vi "Test Data Graph02.vi"() -> ()   [LabVIEW 2020]
uses:
  <vilib>/measure/NI_MABase.lvlib
panel:
  in  "Load":bool
  out "XY":cluster{timestamp[], dbl[]}[](graph)
  in  "P1":dbl(slide) scale=3772664021.7079873..3772664023.307987 scale format="%<%m/%d %H:%M:%S>T"
  in  "P2":dbl(slide) scale=3772664021.7079873..3772664023.307987 scale format="%<%m/%d %H:%M:%S>T"
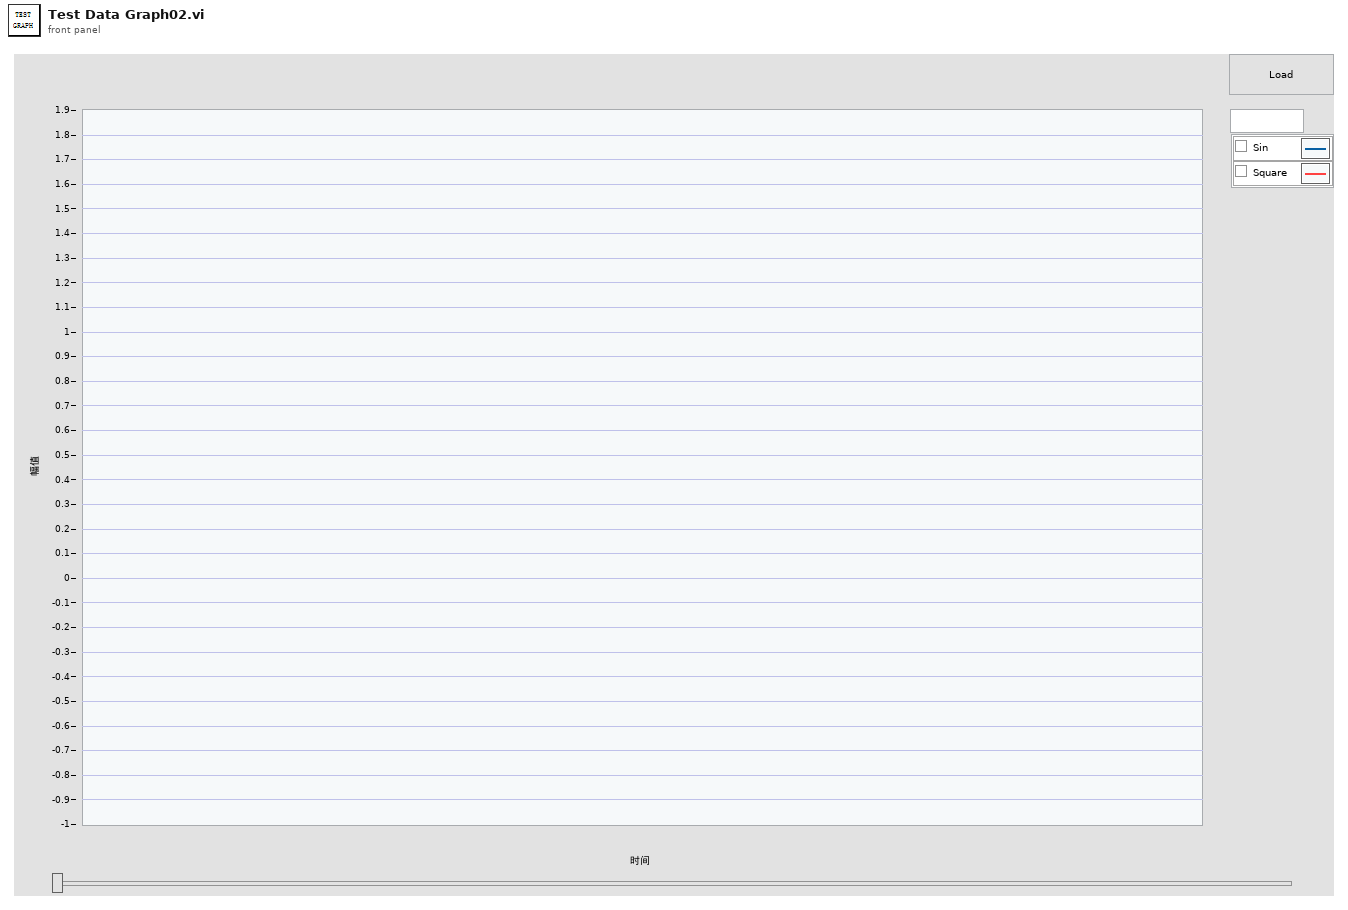
[diagram p1: front panel]
types:
  T1 = cluster{"XY":refnum<vi>, "Maxpoint":i32, "P1":refnum<vi>, "P2":refnum<vi>, "Range":cluster{"IStart":dbl, "CRange":dbl, "IRange":dbl, "CStart":dbl, "Stop":dbl}, "Data":map{string, cluster{"Init":waveform(dbl), "Current":waveform(dbl)}}, "ID":string[]}
  T2 = map{string, cluster{"Init":waveform(dbl), "Current":waveform(dbl)}}
  T3 = cluster{"signal out":waveform(dbl), "signal out":waveform(dbl)}
  T4 = typedef "LVRangeTypeDef.ctl" = cluster{"Minimum":dbl, "Maximum":dbl, "Increment":dbl, "Minor Increment":dbl, "Start":dbl}
  T5 = cluster{"Init":waveform(dbl), "Current":waveform(dbl)}
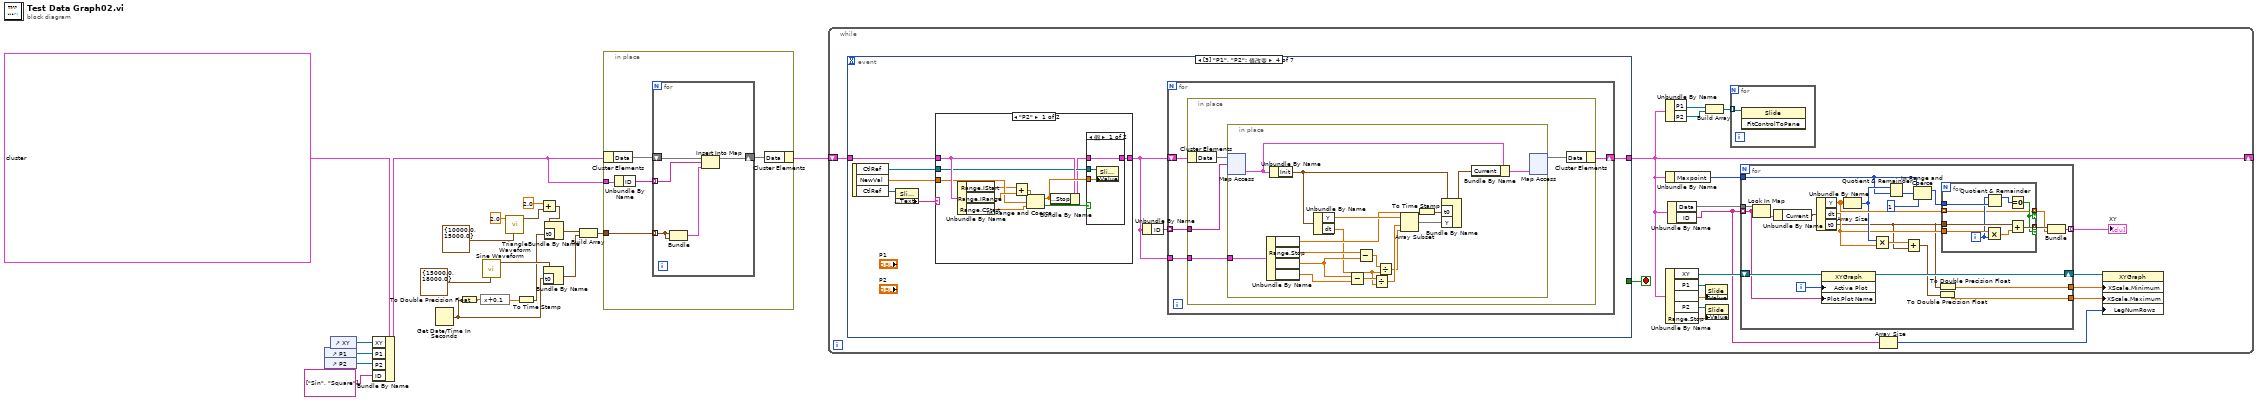
[diagram p0: block diagram]
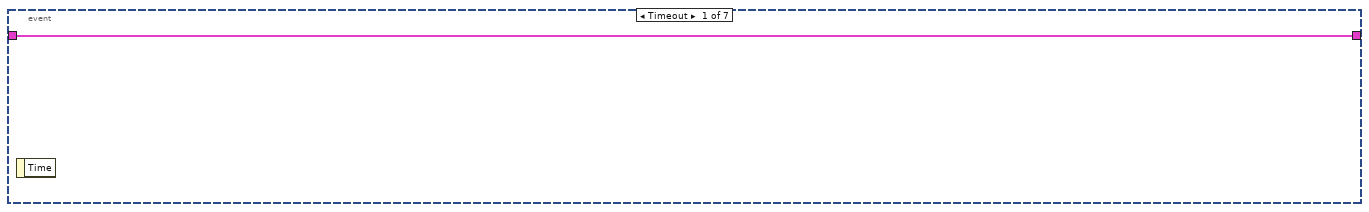
[diagram p2: hidden frame]
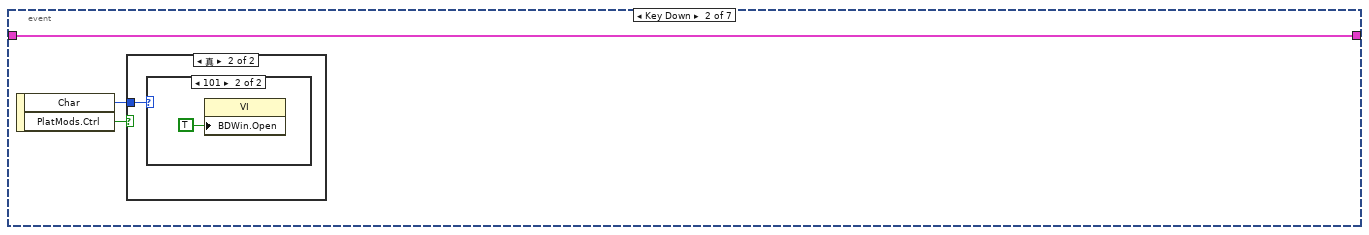
[diagram p3: hidden frame]
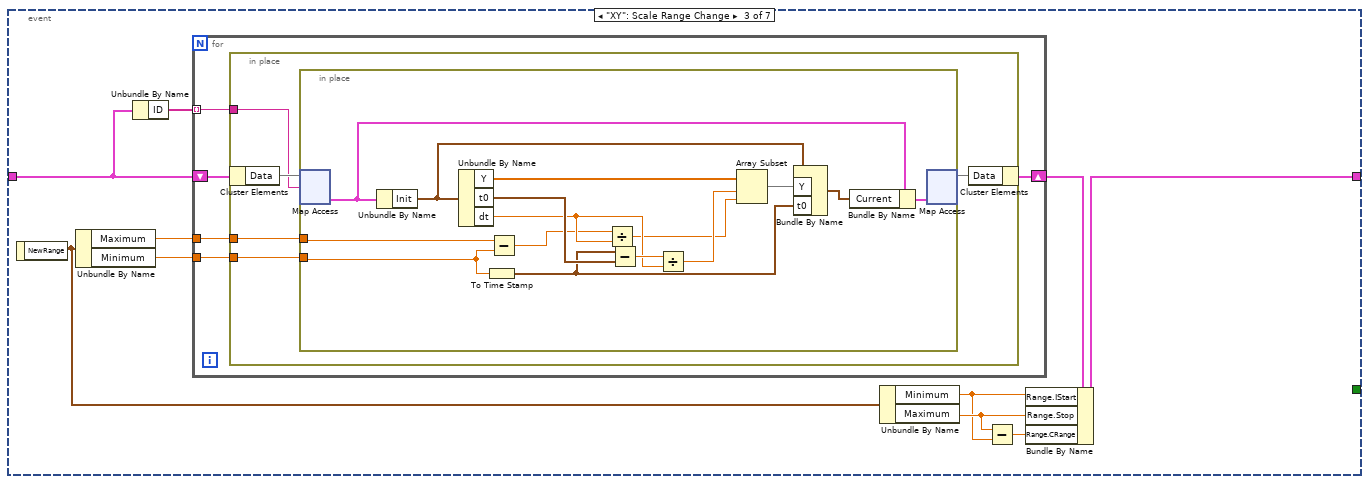
[diagram p6: hidden frame]
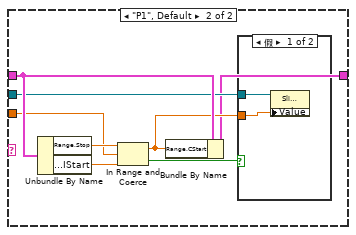
[diagram p8: hidden frame]
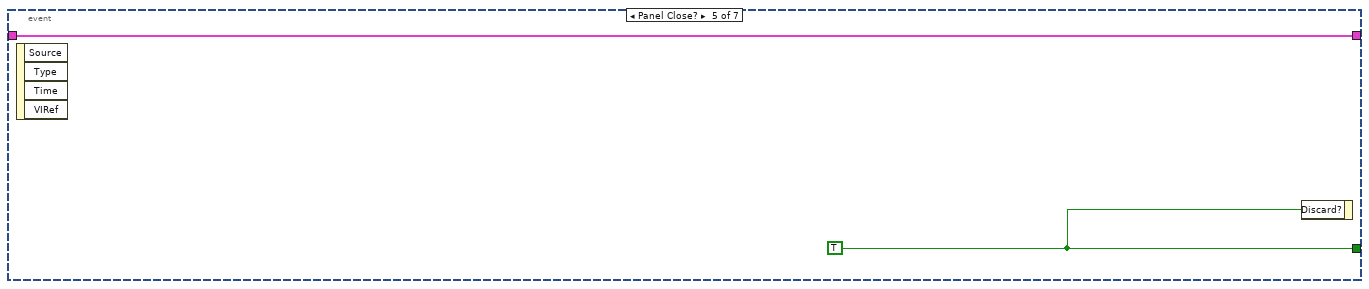
[diagram p10: hidden frame]
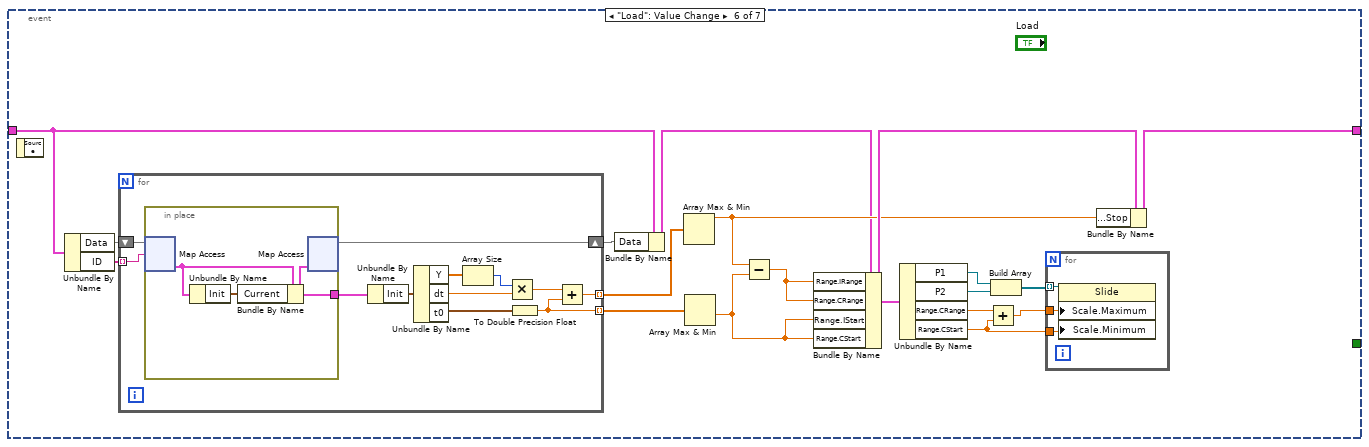
[diagram p11: hidden frame]
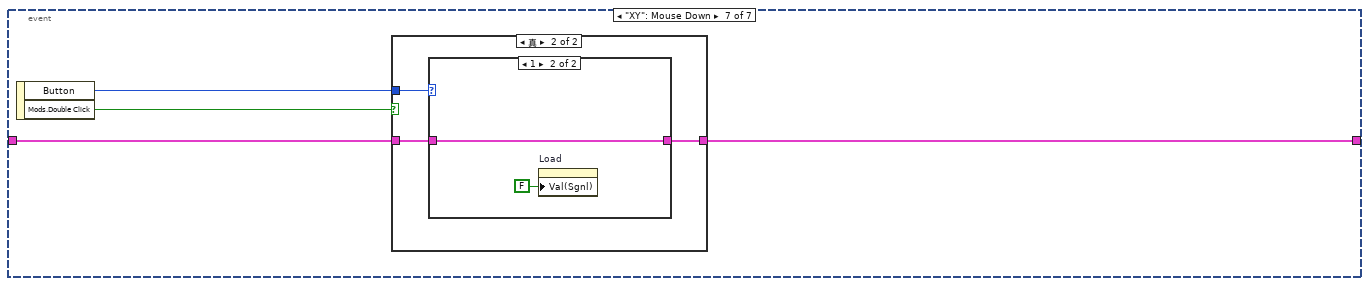
[diagram p12: hidden frame]
diagram:
  n1 = control-ref of="P1"() -> (w19:refnum<vi>)
  n2 = control-ref of="P2"() -> (w18:refnum<vi>)
  n3 = control-ref of="XY"() -> (w20:refnum<vi>)
  n4 = Bundle By Name(cluster=T1 {"XY"=refnum, "Maxpoint"=5000, "P1"=refnum, "P2"=refnum, "Range"={"IStart"=0.0, "CRange"=0.0, "IRange"=0.0, "CStart"=0.0, "Stop"=0.0}, "Data"={}, "ID"=[]}, "XY"=w20, "P1"=w19, "P2"=w18, "ID"=string[] ["Sin", "Square"]) -> (w10:T1)
  n5 = Get Date/Time In Seconds() -> (seconds since 1Jan1904=w3:timestamp)
  n6 = To Double Precision Float(number=w3) -> (double precision float=w16:dbl)
  n7 = expression code="x+0.1"(w16) -> (w17:dbl)
  n8 = call <vilib>:"Sine Waveform.vi"("sampling info"=cluster{"Fs":dbl, "#s":dbl} {"Fs"=15000.0, "#s"=18000.0}) -> ("signal out"=w15:waveform(dbl))  [unwired: 9 in, 1 out]
  n9 = call <vilib>:"Triangle Waveform.vi"("sampling info"=cluster{"Fs":dbl, "#s":dbl} {"Fs"=10000.0, "#s"=15000.0}, "frequency"=2.0) -> ("signal out"=w6:waveform(dbl))  [unwired: 8 in, 1 out]
  n10 = To Time Stamp(1:w17) -> (0:w2:timestamp)
  n11 = Add(x=2.0, y=w6) -> (x+y=w4:waveform(dbl))
  n12 = Bundle By Name(cluster=w15, "t0"=w3) -> (w8:waveform(dbl))
  n13 = Bundle By Name(cluster=w4, "t0"=w2) -> (w9:waveform(dbl))
  n14 = Build Array(w9, w8) -> (w7:waveform(dbl)[])
  n15 = in-place {
    in-place-border: w10 -> [w25]
    in-place-border: w7 -> [w23]
    n16 = in-place-cluster #1(w10) -> ("Data"=w26:T2)
    n17 = Unbundle By Name(w25) -> ("ID"=w24:string[])
    n18 = for {
      shift-right: [w27] -> w22
      shift-left: w26 -> [w31]
      tunnel: w24 -> [w30] mode=indexing
      tunnel: w23 -> [w29] mode=indexing
      n19 = Bundle("signal out"=w29, "signal out"=w29) -> (w28:T3)  [unwired: 1 in]
      n20 = Insert Into Map(map in=w31, key=w30, value=w28) -> (map out=w27:T2)  [unwired: 2 out]
    }
    n21 = in-place-cluster #1("Data"=w22) -> (w12:T1)
  }
  n22 = while {
    shift-right: [w38] -> _
    shift-left: w12 -> [w48]
    stop <- w49 stop-if-true
    n23 = event shown="[3] \"P1\", \"P2\": 值改变" {
      selector: _ -> [_ _ _ _ _ _ _]
      dyn-events: _ -> [_ _ _ _ _ _ _]
      timeout: _ -> [_ _ _ _ _ _ _]
      tunnel: [_ _ _ _ w182 _ _] -> w49
      tunnel: [w82 w83 w96 w128 w181 w194 w219] -> w38
      tunnel: w48 -> [w82 w83 w94 w130 w181 w192 w220]
      event Timeout {
        n24 = event-data() -> ()  [unwired: 1 in, 1 out]
      }
      event Key Down {
        n25 = event-data() -> ("Char"=w85:i16, "PlatMods.Ctrl"=w84:bool)  [unwired: 1 in]
        n26 = case shown="真" w84 {
          tunnel: w85 -> [_ w86]
          frame False {
          }
          frame True {
            n27 = case shown="101" w86 {
              frame 0, Default {
              }
              frame 101 {
                n28 = property class="VI"("BDWin.Open"=TRUE ("程序框图窗口:打开")) -> ()  [unwired: 2 in, 2 out]
              }
            }
          }
        }
      }
      event "XY": Scale Range Change {
        n29 = event-data() -> ("NewRange"=w91:T4)  [unwired: 1 in]
        n30 = Unbundle By Name(w91) -> ("Maximum"=w95:dbl, "Minimum"=w92:dbl)
        n31 = Unbundle By Name(w94) -> ("ID"=w93:string[])
        n32 = for {
          tunnel: w92 -> [w102]
          tunnel: w95 -> [w101]
          shift-right: [w99] -> w97
          shift-left: w94 -> [w100]
          tunnel: w93 -> [w98] mode=indexing
          n33 = in-place {
            in-place-border: w102 -> [w107]
            in-place-border: w101 -> [w106]
            in-place-border: w98 -> [w103]
            n34 = in-place-cluster #2(w100) -> ("Data"=w105:T2)
            n35 = in-place {
              in-place-border: w107 -> [w121]
              in-place-border: w106 -> [w110]
              n36 = in-place-map #3(w105, w103) -> (w109:T5)  [unwired: 1 in, 1 out]
              n37 = Unbundle By Name(w109) -> ("Init"=w114:waveform(dbl))
              n38 = Unbundle By Name(w114) -> ("Y"=w120:dbl[], "t0"=w122:timestamp, "dt"=w117:dbl)
              n39 = To Time Stamp(1:w121) -> (0:w112:timestamp)
              n40 = Subtract(x=w110, y=w121) -> (x-y=w111:dbl)
              n41 = Divide(x=w111, y=w117) -> (x/y=w115:dbl)
              n42 = Subtract(x=w112, y=w122) -> (x-y=w118:dbl)
              n43 = Divide(x=w118, y=w117) -> (x/y=w116:dbl)
              n44 = Array Subset(array=w120, index=w116, length=w115) -> (w119:dbl[])
              n45 = Bundle By Name(cluster=w114, "Y"=w119, "t0"=w112) -> (w113:waveform(dbl))
              n46 = Bundle By Name(cluster=w109, "Current"=w113) -> (w108:T5)
              n47 = in-place-map #3(w108) -> (w104:T2)  [unwired: 1 in, 2 out]
            }
            n48 = in-place-cluster #2("Data"=w104) -> (w99:T1)
          }
        }
        n49 = Unbundle By Name(w91) -> ("Minimum"=w89:dbl, "Maximum"=w90:dbl)
        n50 = Subtract(x=w90, y=w89) -> (x-y=w88:dbl)
        n51 = Bundle By Name(cluster=w97, "Range.IStart"=w89, "Range.Stop"=w90, "Range.CRange"=w88) -> (w96:T1)
      }
      event "P1", "P2": Value Change {
        n52 = event-data() -> ("CtlRef"=w125:refnum<vi>, "NewVal"=w129:dbl, "CtlRef"=w127:refnum<vi>)  [unwired: 1 in]
        n53 = property class="Slide (严格)"(reference=w127) -> ("Label.Text"=w126:string)  [unwired: 1 in, 2 out]
        n54 = case shown="\"P2\"" w126 {
          tunnel: w130 -> [w161 w178]
          tunnel: w129 -> [w159 w176]
          tunnel: w125 -> [w160 w174]
          tunnel: [w162 w171] -> w123
          frame "P2" {
            n55 = Unbundle By Name(w161) -> ("Range.IStart"=w157:dbl, "Range.IRange"=w164:dbl, "Range.CStart"=w156:dbl)
            n56 = Add(x=w157, y=w164) -> (x+y=w163:dbl)
            n57 = In Range and Coerce(upper limit=w163, x=w159, lower limit=w156) -> (coerced(x)=w166:dbl, In Range?=w165:bool)
            n58 = Bundle By Name(cluster=w161, "Range.Stop"=w166) -> (w158:T1)
            n59 = case shown="假" w165 {
              tunnel: w158 -> [w168 w170]
              tunnel: w166 -> [w169 _]
              tunnel: [w168 w170] -> w162
              tunnel: w160 -> [w167 _]
              frame False {
                n60 = property class="Slide (严格)"(reference=w167, "Value"=w169) -> ()  [unwired: 1 in, 2 out]
              }
              frame True {
              }
            }
          }
          frame "P1", Default {
            n61 = Unbundle By Name(w178) -> ("Range.Stop"=w177:dbl, "Range.IStart"=w175:dbl)
            n62 = In Range and Coerce(upper limit=w177, x=w176, lower limit=w175) -> (coerced(x)=w173:dbl, In Range?=w172:bool)
            n63 = Bundle By Name(cluster=w178, "Range.CStart"=w173) -> (w171:T1)
            n64 = case shown="假" w172 {
              tunnel: w174 -> [w180 _]
              tunnel: w173 -> [w179 _]
              frame False {
                n65 = property class="Slide (严格)"(reference=w180, "Value"=w179) -> ()  [unwired: 1 in, 2 out]
              }
              frame True {
              }
            }
          }
        }
        n66 = Unbundle By Name(w123) -> ("ID"=w124:string[])
        n67 = for {
          shift-right: [w132] -> w128
          shift-left: w123 -> [w134]
          tunnel: w124 -> [w133] mode=indexing
          tunnel: w123 -> [w131]
          n68 = in-place {
            in-place-border: w133 -> [w136]
            in-place-border: w131 -> [w135]
            n69 = in-place-cluster #4(w134) -> ("Data"=w138:T2)
            n70 = in-place {
              in-place-border: w135 -> [w139]
              n71 = in-place-map #5(w138, w136) -> (w141:T5)  [unwired: 1 in, 1 out]
              n72 = Unbundle By Name(w139) -> ("Range.CStart"=w144:dbl, "Range.Stop"=w153:dbl, "Range.CStart"=w143:dbl, "Range.IStart"=w149:dbl)
              n73 = Unbundle By Name(w141) -> ("Init"=w152:waveform(dbl))
              n74 = Unbundle By Name(w152) -> ("Y"=w150:dbl[], "dt"=w142:dbl)
              n75 = Subtract(x=w143, y=w149) -> (x-y=w148:dbl)
              n76 = Subtract(x=w153, y=w143) -> (x-y=w151:dbl)
              n77 = Divide(x=w148, y=w142) -> (x/y=w146:dbl)
              n78 = Divide(x=w151, y=w142) -> (x/y=w145:dbl)
              n79 = Array Subset(array=w150, index=w146, length=w145) -> (w147:dbl[])
              n80 = To Time Stamp(1:w144) -> (0:w155:timestamp)
              n81 = Bundle By Name(cluster=w152, "t0"=w155, "Y"=w147) -> (w154:waveform(dbl))
              n82 = Bundle By Name(cluster=w141, "Current"=w154) -> (w140:T5)
              n83 = in-place-map #5(w140) -> (w137:T2)  [unwired: 1 in, 2 out]
            }
            n84 = in-place-cluster #4("Data"=w137) -> (w132:T1)
          }
        }
      }
      event Panel Close? {
        w182 = TRUE ("放弃？")
        n85 = event-data() -> ()  [unwired: 1 in, 4 out]
        n86 = event-data("Discard?"=w182) -> ()  [unwired: 1 in, 1 out]
      }
      event "Load": Value Change {
        n87 = event-data() -> ()  [unwired: 1 in, 1 out]
        n88 = Unbundle By Name(w192) -> ("Data"=w185:T2, "ID"=w191:string[])
        n89 = for {
          tunnel: w191 -> [w204] mode=indexing
          tunnel: [w206] -> w189 mode=indexing
          tunnel: [w205] -> w190 mode=indexing
          shift-right: [w202] -> w183
          shift-left: w185 -> [w203]
          n90 = in-place {
            in-place-border: [w213] -> w201
            n91 = in-place-map #6(w203, w204) -> (w215:T5)  [unwired: 1 in, 1 out]
            n92 = Unbundle By Name(w215) -> ("Init"=w214:waveform(dbl))
            n93 = Bundle By Name(cluster=w215, "Current"=w214) -> (w213:T5)
            n94 = in-place-map #6(w213) -> (w202:T2)  [unwired: 1 in, 2 out]
          }
          n95 = Unbundle By Name(w201) -> ("Init"=w208:waveform(dbl))
          n96 = Unbundle By Name(w208) -> ("Y"=w211:dbl[], "dt"=w210:dbl, "t0"=w209:timestamp)
          n97 = Array Size(array=w211) -> (size(s)=w212:i32)
          n98 = Multiply(x=w212, y=w210) -> (x*y=w207:dbl)
          n99 = To Double Precision Float(number=w209) -> (double precision float=w206:dbl)
          n100 = Add(x=w207, y=w206) -> (x+y=w205:dbl)
        }
        n101 = Bundle By Name(cluster=w192, "Data"=w183) -> (w184:T1)
        n102 = Array Max & Min(array=w190) -> (max value=w187:dbl)  [unwired: 3 out]
        n103 = Array Max & Min(array=w189) -> (min value=w188:dbl)  [unwired: 3 out]
        n104 = Subtract(x=w187, y=w188) -> (x-y=w186:dbl)
        n105 = Bundle By Name(cluster=w184, "Range.IRange"=w186, "Range.CRange"=w186, "Range.IStart"=w188, "Range.CStart"=w188) -> (w196:T1)
        n106 = Unbundle By Name(w196) -> ("P1"=w199:refnum<vi>, "P2"=w198:refnum<vi>, "Range.CRange"=w197:dbl, "Range.CStart"=w195:dbl)
        n107 = Add(x=w197, y=w195) -> (x+y=w193:dbl)
        n108 = Build Array(w199, w198) -> (w200:refnum<vi>[])
        n109 = for {
          tunnel: w200 -> [w218] mode=indexing
          tunnel: w193 -> [w217]
          tunnel: w195 -> [w216]
          n110 = property class="Slide"(reference=w218, "Scale.Maximum"=w217, "Scale.Minimum"=w216) -> ()  [unwired: 1 in, 2 out]
        }
        n111 = Bundle By Name(cluster=w196, "Range.Stop"=w187) -> (w194:T1)
      }
      event "XY": Mouse Down {
        n112 = event-data() -> ("Button"=w221:u16, "Mods.Double Click"=w222:bool)  [unwired: 1 in]
        n113 = case shown="真" w222 {
          tunnel: w221 -> [_ w226]
          tunnel: [w223 w225] -> w219
          tunnel: w220 -> [w223 w224]
          frame False {
          }
          frame True {
            n114 = case shown="1" w226 {
              tunnel: [w227 w229] -> w225
              tunnel: w224 -> [w227 w229]
              frame 0, Default {
              }
              frame 1 {
                n115 = property on="Load" class="Bool (严格)"("Val(Sgnl)"=FALSE ("值(信号)")) -> ()  [unwired: 2 in, 2 out]
              }
            }
          }
        }
      }
    }
    n116 = Unbundle By Name(w38) -> ("P1"=w39:refnum<vi>, "P2"=w40:refnum<vi>)
    n117 = Unbundle By Name(w38) -> ("Maxpoint"=w45:i32)
    n118 = Unbundle By Name(w38) -> ("XY"=w34:refnum<vi>, "P1"=w44:refnum<vi>, "Range.CStart"=w42:dbl, "P2"=w43:refnum<vi>, "Range.Stop"=w37:dbl)
    n119 = Unbundle By Name(w38) -> ("Data"=w35:T2, "ID"=w33:string[])
    n120 = Build Array(w39, w40) -> (w41:refnum<vi>[])
    n121 = property class="Slide"(reference=w44, "Value"=w42) -> ()  [unwired: 1 in, 2 out]
    n122 = property class="Slide"(reference=w43, "Value"=w37) -> ()  [unwired: 1 in, 2 out]
    n123 = for {
      tunnel: w41 -> [w81] mode=indexing
      n124 = invoke class="Slide" method="FitControlToPane"(reference=w81) -> ()  [unwired: 2 in, 3 out]
    }
    n125 = for {
      tunnel: [w63] -> w47
      tunnel: [w61] -> w46
      tunnel: w45 -> [w59]
      tunnel: [w57] -> w36 mode=indexing
      tunnel: w33 -> [w50] mode=indexing
      tunnel: w35 -> [w56]
      shift-right: [w52] -> _
      shift-left: w34 -> [w53]
      i -> [w51]
      n126 = Look In Map(map=w56, key=w50) -> (value=w55:T5)  [unwired: 1 in, 1 out]
      n127 = Unbundle By Name(w55) -> ("Current"=w54:waveform(dbl))
      n128 = Unbundle By Name(w54) -> ("Y"=w71:dbl[], "dt"=w65:dbl, "t0"=w60:timestamp)
      n129 = property class="XYGraph"(reference=w53, "Active Plot"=w51, "Plot.Plot Name"=w50) -> (reference out=w52:refnum<vi>)  [unwired: 1 in, 1 out]
      n130 = Array Size(array=w71) -> (size(s)=w66:i32)
      n131 = Multiply(x=w66, y=w65) -> (x*y=w64:dbl)
      n132 = Quotient & Remainder(x=w66, y=w59) -> (floor(x/y)=w68:i32)  [unwired: 1 out]
      n133 = Add(x=w64, y=w60) -> (x+y=w62:timestamp)
      n134 = In Range and Coerce(upper limit=w59, x=w68, lower limit=1 ("下限")) -> (coerced(x)=w67:i32)  [unwired: 1 out]
      n135 = To Double Precision Float(number=w62) -> (double precision float=w61:dbl)
      n136 = To Double Precision Float(number=w60) -> (double precision float=w63:dbl)
      n137 = for {
        tunnel: w71 -> [w72] mode=indexing
        tunnel: w60 -> [w80]
        tunnel: w65 -> [w79]
        tunnel: [w77] -> w70 mode=indexing if=w76
        tunnel: [w72] -> w58 mode=indexing if=w76
        tunnel: w67 -> [w74]
        i -> [w73]
        n138 = Multiply(x=w79, y=w73) -> (x*y=w78:dbl)
        n139 = Quotient & Remainder(x=w73, y=w74) -> (x-y*floor(x/y)=w75:i32)  [unwired: 1 out]
        n140 = Equal To 0?(x=w75) -> (x = 0?=w76:bool)
        n141 = Add(x=w80, y=w78) -> (x+y=w77:timestamp)
      }
      n142 = Bundle(w70, w58) -> (w57:cluster{timestamp[], dbl[]})  [unwired: 1 in]
    }
    "XY" <- w36
    n143 = Array Size(array=w33) -> (size(s)=w32:i32)
    n144 = property on="属性节点" class="XYGraph"(reference=w34, "XScale.Minimum"=w47, "XScale.Maximum"=w46, "LegNumRows"=w32) -> ()  [unwired: 1 in, 2 out]
  }
